vi "U3 2-PWM.vi"(8 "error in":errorcluster, 9 "Timer0 Duty Cycle [%]":dbl=50.0 format="%.1f", 10 "16-bit PWM Frequency [Hz]":dbl=40.0 format="%.2f") -> (2 "Actual 16-bit Frequency":dbl format="%.1f")   [LabVIEW 2021]
panel:
  in  "Timer/Counter Pin Offset":u8
  out "Update":bool
  out "Timer Value Array":u16[](array[numeric])
  in  "Timer1 Duty Cycle [%]":dbl=50.0 format="%.1f"
  in  "stop":bool
  out "Actual 8-bit Frequency":dbl format="%.1f"
  in  "FirstFound":bool=TRUE
  in  "Address":string="1"
  out "TimerClockDivisor":u8
  out "Error Message":string
  # "Demonstrates 1 channel of 16-bit PWM output and 1 channel of 8-bit PWM output.\nUses the 24 MHz divisor capable clock, and chooses a timer clock divisor to get\nas close as possible to the desired 16-bit PWM frequency.  Since a divisor capable\nclock is used, Counter1 is not available.  Since all timers use the same clock, the\nfrequency of the 8-bit PWM is fixed at 256 times the frequency of the 16-bit PWM."
  # "Range is 1.43 to 366.21 Hz"
  # "This example allows the duty cycles to\nbe changed while the VI is running."
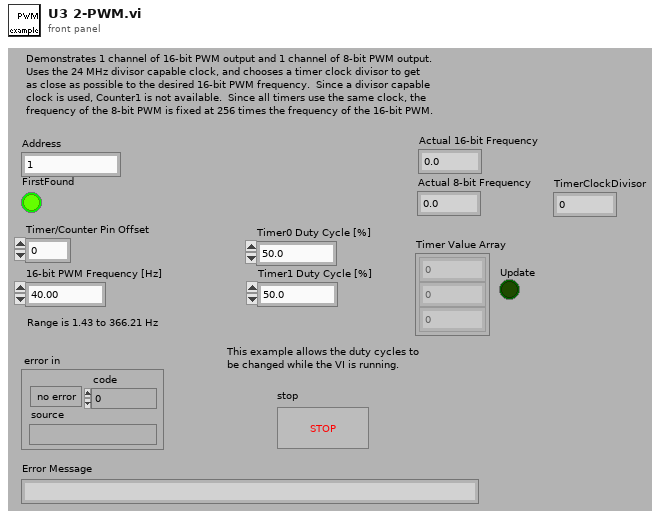
[diagram p1: front panel]
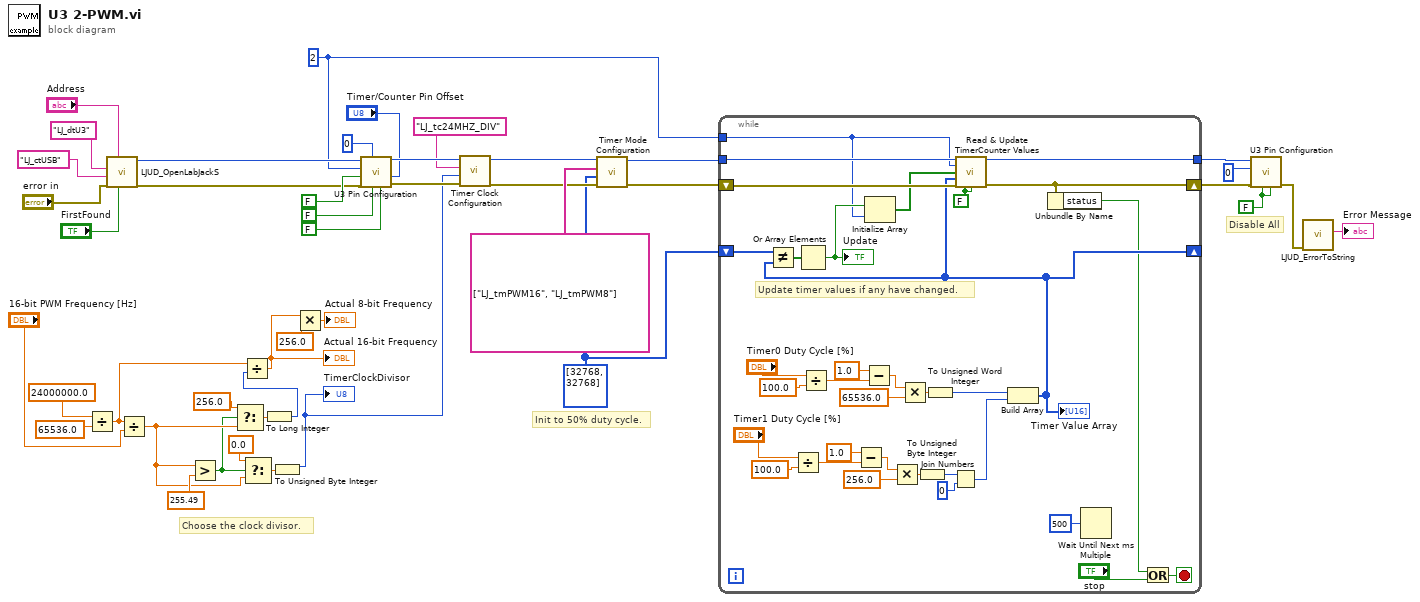
[diagram p0: block diagram]
diagram:
  w1 = u8 2 ("Number of Timers Enabled")
  w27 = FALSE ("Enable Counter0")
  w8 = u16[] [32768, 32768] ("TimerValues")
  # "Disable All"
  # "Choose the clock divisor."
  # "Init to 50% duty cycle."
  n1 = Divide(x=24000000.0, y=65536.0) -> (x/y=w31:dbl)
  n2 = call "LJUD_OpenLabJackS.vi"("FirstFound"="FirstFound", "Address"="Address", "error in"="error in", "ConnectionType"="LJ_ctUSB", "DeviceType"="LJ_dtU3") -> ("error out"=w11:errorcluster, "Handle"=w12:i32)  [unwired: 4 in, 1 out]
  n3 = Divide(x=w31, y="16-bit PWM Frequency [Hz]") -> (x/y=w35:dbl)
  n4 = Greater?(x=w35, y=255.49) -> (0:w34:bool)
  n5 = Select(t=256.0, s=w34, f=w35) -> (s? t:f=w37:dbl)
  n6 = Select(t=0.0, s=w34, f=w35) -> (s? t:f=w40:dbl)
  n7 = To Long Integer(number=w37) -> (32bit integer=w33:i32)
  n8 = Divide(x=w31, y=w33) -> (x/y=w30:dbl)
  "Actual 16-bit Frequency" <- w30
  n9 = To Unsigned Byte Integer(number=w40) -> (unsigned 8bit integer=w9:u8)
  "TimerClockDivisor" <- w9
  n10 = Multiply(x=w30, y=256.0) -> (x*y=→"Actual 8-bit Frequency":dbl)
  n11 = call "U3 Pin Configuration.vi"("Timer/Counter Pin Offset"="Timer/Counter Pin Offset", "Enable Counter1"=FALSE ("Enable Counter0"), "Enable Counter0"=FALSE, "FIO/EIO Analog Enable"=0, "error in"=w11, "Enable DAC1"=FALSE ("Enable Counter0"), "Number of Timers Enabled"=w1, "Handle In"=w12) -> ("error out"=w19:errorcluster, "Handle Out"=w18:i32)  [unwired: 2 in]
  n12 = call "Timer Clock Configuration.vi"("error in"=w19, "Timer Clock Divisor"=w9, "Timer Clock Base"="LJ_tc24MHZ_DIV", "Handle In"=w18) -> ("error out"=w20:errorcluster, "Handle Out"=w17:i32)  [unwired: 6 in]
  n13 = call "Timer Mode Configuration.vi"("error in"=w20, "TimerValues"=w8, "TimerModes"=string[] ["LJ_tmPWM16", "LJ_tmPWM8"], "Handle In"=w17) -> ("error out"=w13:errorcluster, "Handle Out"=w14:i32)  [unwired: 6 in]
  n14 = while {
    shift-right: [w58] -> w25
    shift-left: w13 -> [w61]
    tunnel: w14 -> [w60]
    shift-right: [w52] -> _
    shift-left: w8 -> [w57]
    tunnel: [w53] -> w26
    tunnel: w1 -> [w46]
    stop <- w59 stop-if-true
    w45 = FALSE ("Reset Counter0")
    # "Update timer values if any have changed."
    n15 = Divide(x="Timer1 Duty Cycle [%]", y=100.0) -> (x/y=w75:dbl)
    n16 = Divide(x="Timer0 Duty Cycle [%]", y=100.0) -> (x/y=w67:dbl)
    n17 = Subtract(x=1.0, y=w75) -> (x-y=w73:dbl)
    n18 = Subtract(x=1.0, y=w67) -> (x-y=w65:dbl)
    n19 = Multiply(x=w73, y=256.0) -> (x*y=w70:dbl)
    n20 = Multiply(x=w65, y=65536.0) -> (x*y=w64:dbl)
    n21 = To Unsigned Byte Integer(number=w70) -> (unsigned 8bit integer=w72:u8)
    n22 = To Unsigned Word Integer(number=w64) -> (unsigned 16bit integer=w62:u16)
    n23 = Join Numbers(hi=w72, lo=u8 0) -> ((hi.lo)=w47:u16)
    n24 = Build Array(w62, w47) -> (w52:u16[])
    "Timer Value Array" <- w52
    n25 = Not Equal?(x=w57, y=w52) -> (x != y?=w56:bool[])
    n26 = Or Array Elements(Boolean array=w56) -> (logical OR=w55:bool)
    "Update" <- w55
    n27 = Initialize Array(w55, w46) -> (w54:bool[])
    n28 = call "Read & Update TimerCounter Values.vi"("Handle In"=w60, "# Timers to Read"=w46, "UpdateReset Timers"=w54, "TimerValues"=w52, "error in"=w61, "Read Counter0"=w45, "Read Counter1"=w45) -> ("Handle Out"=w53:i32, "error out"=w58:errorcluster)  [unwired: 5 in, 2 out]
    n29 = Unbundle By Name(w58) -> ("status"=w51:bool)
    n30 = Wait Until Next ms Multiple(millisecond multiple=u32 500) -> ()  [unwired: 1 out]
    n31 = Or(x=w51, y="stop") -> (x .or. y?=w59:bool)
  }
  n32 = call "U3 Pin Configuration.vi"("Enable Counter1"=w27, "Enable Counter0"=w27, "error in"=w25, "Number of Timers Enabled"=u8 0 ("# Timers Enabled"), "Handle In"=w26) -> ("error out"=w24:errorcluster)  [unwired: 5 in, 1 out]
  n33 = call "LJUD_ErrorToString.vi"("error in"=w24) -> ("String"=→"Error Message":string)  [unwired: 10 in]
